vi "Main_NumberGenerator.vi"() -> ()   [LabVIEW 2018]
uses:
  <vilib>/Platform/browser.llb/Open URL in Default Browser (string).vi
panel:
  in  "ABRIR BARCODE":bool
  in  "Information Tool":bool
  in  "LIMPIAR":bool
  in  "SALIR":bool
  out "Numero seleccionado":string
  in  "Numeros generados":i32(listbox)
  in  "NumerosAGenerar":i32
  in  "Generar":bool
  # "Numeros a generar"
  # "Developed by: Juan Pablo Aldape Aranda"
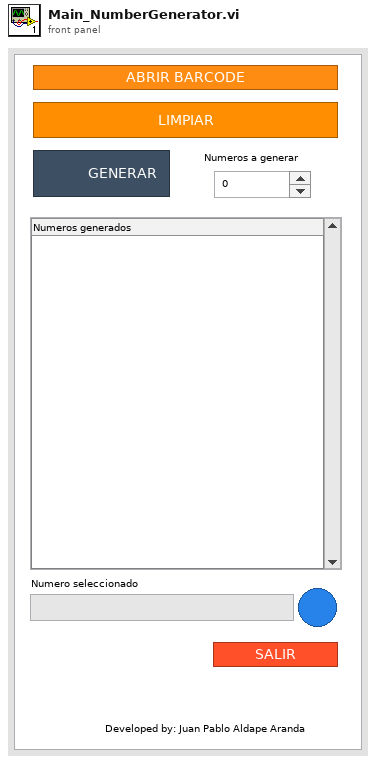
[diagram p1: front panel]
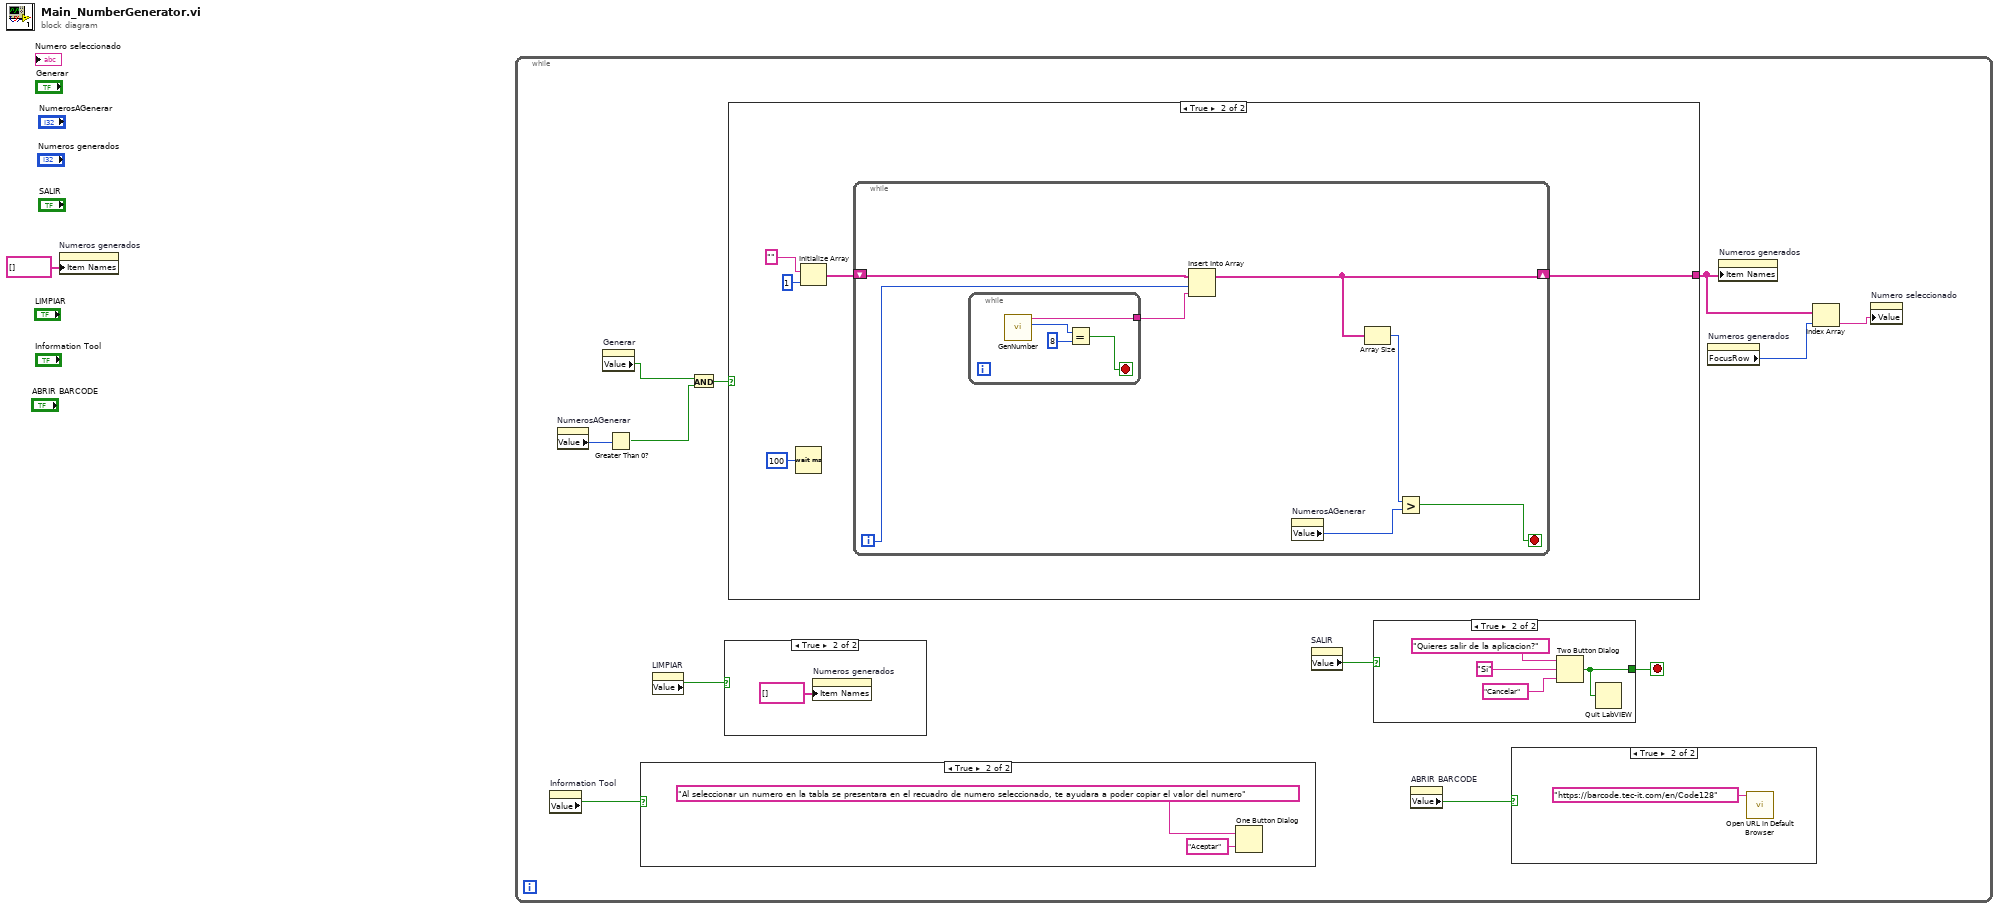
[diagram p0: block diagram]
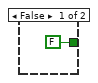
[diagram p5: hidden frame]
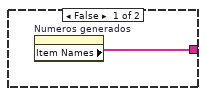
[diagram p6: hidden frame]
diagram:
  n1 = property on="Numeros generados" class="LstBox (strict)"("Item Names"=string[] []) -> ()  [unwired: 2 in, 2 out]
  n2 = while {
    stop <- w9 stop-if-true
    n3 = property on="Information Tool" class="Bool (strict)"() -> ("Value"=w3:bool)  [unwired: 2 in, 2 out]
    n4 = property on="NumerosAGenerar" class="DigNum (strict)"() -> ("Value"=w8:i32)  [unwired: 2 in, 2 out]
    n5 = property on="Generar" class="Bool (strict)"() -> ("Value"=w7:bool)  [unwired: 2 in, 2 out]
    n6 = Greater Than 0?(x=w8) -> (x > 0?=w6:bool)
    n7 = case shown="True" w3 {
      frame False {
      }
      frame True {
        n8 = One Button Dialog(message="Al seleccionar un numero en la tabla se presentara en el recuadro de numero seleccionado, te ayudara a poder copiar el valor del numero", button name ("OK")="Aceptar") -> ()  [unwired: 1 out]
      }
    }
    n9 = property on="LIMPIAR" class="Bool (strict)"() -> ("Value"=w4:bool)  [unwired: 2 in, 2 out]
    n10 = And(x=w7, y=w6) -> (x .and. y?=w5:bool)
    n11 = case shown="True" w4 {
      frame False {
      }
      frame True {
        n12 = property on="Numeros generados" class="LstBox (strict)"("Item Names"=string[] []) -> ()  [unwired: 2 in, 2 out]
      }
    }
    n13 = case shown="True" w5 {
      tunnel: [w23 w25] -> w13
      frame False {
        n14 = property on="Numeros generados" class="LstBox (strict)"() -> ("Item Names"=w23:string[])  [unwired: 2 in, 2 out]
      }
      frame True {
        n15 = Wait (ms)(milliseconds to wait=u32 100) -> ()  [unwired: 1 out]
        n16 = Initialize Array("", 1 ("dimension size")) -> (w26:string[])
        n17 = while {
          shift-right: [w31] -> w25
          shift-left: w26 -> [w33]
          i -> [w29]
          stop <- w34 stop-if-true
          n18 = while {
            tunnel: [w36] -> w32
            stop <- w37 stop-if-true
            n19 = call "GenNumber.vi"() -> ("LongitudDelNumero"=w39:i32, "RandoNumber"=w36:string)  [unwired: 10 in]
            n20 = Equal?(x=w39, y=8) -> (x = y?=w37:bool)
          }
          n21 = Insert Into Array(array=w33, index=w29, new element=w32) -> (w31:string[])
          n22 = property on="NumerosAGenerar" class="DigNum (strict)"() -> ("Value"=w35:i32)  [unwired: 2 in, 2 out]
          n23 = Array Size(array=w31) -> (size(s)=w30:i32)
          n24 = Greater?(x=w30, y=w35) -> (0:w34:bool)
        }
      }
    }
    n25 = property on="SALIR" class="Bool (strict)"() -> ("Value"=w10:bool)  [unwired: 2 in, 2 out]
    n26 = case shown="True" w10 {
      tunnel: [FALSE ("T button?") w19] -> w9
      frame False {
      }
      frame True {
        n27 = Two Button Dialog(message="Quieres salir de la aplicacion?", 1:"Cancelar" ("F button name (\"Cancel\")"), 2:"Si" ("T button name (\"OK\")")) -> (T button?=w19:bool)
        n28 = Quit LabVIEW(quit? (T)=w19) -> ()
      }
    }
    n29 = property on="ABRIR BARCODE" class="Bool (strict)"() -> ("Value"=w2:bool)  [unwired: 2 in, 2 out]
    n30 = case shown="True" w2 {
      frame False {
      }
      frame True {
        n31 = call-poly <vilib>:"Open URL in Default Browser.vi"("URL"="https://barcode.tec-it.com/en/Code128") -> ()  [unwired: 5 in, 2 out]
      }
    }
    n32 = property on="Numeros generados" class="LstBox (strict)"() -> ("FocusRow"=w12:i32)  [unwired: 2 in, 2 out]
    n33 = property on="Numeros generados" class="LstBox (strict)"("Item Names"=w13) -> ()  [unwired: 2 in, 2 out]
    n34 = Index Array(array=w13, index=w12) -> (element=w11:string)
    n35 = property on="Numero seleccionado" class="Str"("Value"=w11) -> ()  [unwired: 2 in, 2 out]
  }
